vi "Swerve_Simple Config.vi"(11 "Module Azimuth Config Data":T7) -> (0 "PhoenixMotorControlDevRef Out":T2, 1 "PhoenixMotorControlDevRef Out":T2, 2 "CTRE_CANcoder_DeviceRef Out":T1, 3 "Motor Pos Out":T8)   [LabVIEW 2023, in "Thor-SwerveDrive_ACT.lvlib"]
uses:
  Thor-SwerveDrive_ACT.lvlib
  <vilib>/Rock Robotics/WPI/ThirdParty/Phoenix-LabVIEW/CANCoder/Set/CTRE_Phoenix_CANcoder_SetPositionToAbsolute.vi
  Shared Code/TypeDefs/ENUM_Motor Index.ctl
  Shared Code/TypeDefs/Cluster_Module Specific Config Data.ctl
  <vilib>/Rock Robotics/SystemInterfaces/DIO/FPGA_DIOPWMChannel.ctl
  <vilib>/Rock Robotics/WPI/PWM/WPI_PWMDeadband.ctl
  <vilib>/Rock Robotics/WPI/MotorControl/WPI_MotorControlType.ctl
  <vilib>/Rock Robotics/SystemInterfaces/DIO/FPGA_DIOChannel.ctl
  <vilib>/Rock Robotics/WPI/MotorControl/WPI_MotorControlDeviceRef.ctl
  <vilib>/Rock Robotics/WPI/ThirdParty/Phoenix-LabVIEW/CANCoder/Controls/CTRE_Phoenix_CANcoder_DeviceRef.ctl
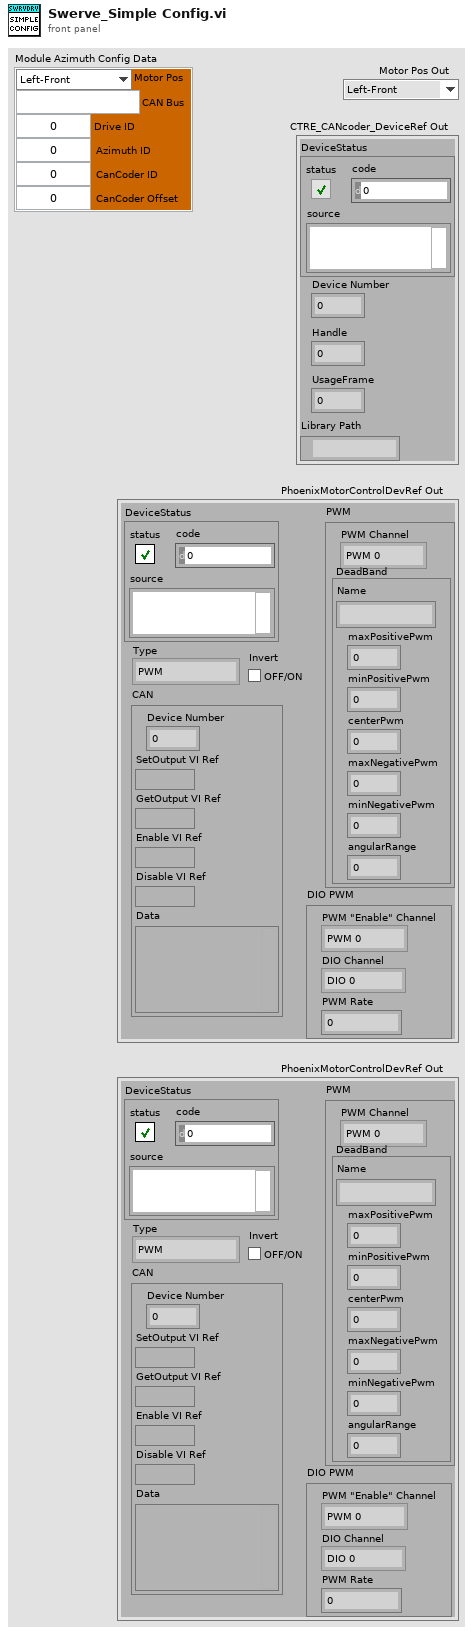
[diagram p1: front panel]
types:
  T1 = typedef "CTRE_Phoenix_CANcoder_DeviceRef.ctl" = cluster{"DeviceStatus":errorcluster, "Device Number":u8, "Handle":u64, "UsageFrame":u32, "Library Path":path}
  T2 = typedef "WPI_MotorControlDeviceRef.ctl" = cluster{"DeviceStatus":errorcluster, "Type":T3, "PWM":cluster{"PWM Channel":T4, "DeadBand":T5}, "CAN":cluster{"Device Number":u8, "SetOutput VI Ref":variant, "GetOutput VI Ref":variant, "Enable VI Ref":variant, "Disable VI Ref":variant, "Data":variant}, "Invert":bool, "DIO PWM":cluster{"PWM \"Enable\" Channel":T4, "DIOChannel":T6, "PWM Rate":dbl}}
  T3 = typedef "WPI_MotorControlType.ctl" = enum16{"PWM", "CAN", "DIO PWM"}
  T4 = typedef "FPGA_DIOPWMChannel.ctl" = enum8{"PWM 0", "PWM 1", "PWM 2", "PWM 3", "PWM 4", "PWM 5", "PWM 6", "PWM 7", "PWM 8", "PWM 9", "PWM MXP 0", "PWM MXP 1", "PWM MXP 2", "PWM MXP 3", "PWM MXP 4", "PWM MXP 5", "PWM MXP 6", "PWM MXP 7", "PWM MXP 8", "PWM MXP 9", "Invalid"}
  T5 = typedef "WPI_PWMDeadband.ctl" = cluster{"Name":string, "maxPositivePwm":i32, "minPositivePwm":i32, "centerPwm":i32, "maxNegativePwm":i32, "minNegativePwm":i32, "angularRange":u16}
  T6 = typedef "FPGA_DIOChannel.ctl" = enum8{"DIO 0", "DIO 1", "DIO 2", "DIO 3", "DIO 4", "DIO 5", "DIO 6", "DIO 7", "DIO 8", "DIO 9", "DIO MXP 0", "DIO MXP 1", "DIO MXP 2", "DIO MXP 3", "DIO MXP 4", "DIO MXP 5", "DIO MXP 6", "DIO MXP 7", "DIO MXP 8", "DIO MXP 9", "DIO MXP 10", "DIO MXP 11", "DIO MXP 12", "DIO MXP 13", "DIO MXP 14", "DIO MXP 15", "SPI Port CS1", "SPI Port CS2", "SPI Port CS3", "SPI Port MISO", "SPI Port MOSI", "Invalid"}
  T7 = typedef "Cluster_Module Specific Config Data.ctl" = cluster{"Motor Pos":T8, "CAN Bus":string, "Drive ID":u8, "Azimuth ID":u8, "CanCoder ID":u8, "CanCoder Offset":dbl}
  T8 = typedef "ENUM_Motor Index.ctl" = enum16{"Left-Front", "Right-Front", "Left-Back", "Right-Back"}
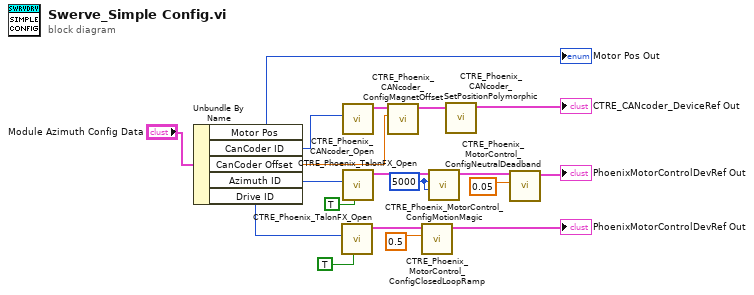
[diagram p0: block diagram]
diagram:
  w8 = 5000 ("Cruise Velocity")
  n1 = Unbundle By Name("Module Azimuth Config Data") -> ("Motor Pos"=→"Motor Pos Out":T8, "CanCoder ID"=w16:u8, "CanCoder Offset"=w1:dbl, "Azimuth ID"=w17:u8, "Drive ID"=w18:u8)
  n2 = call <vilib>:"CTRE_Phoenix_TalonFX_Open.vi"("Invert"=TRUE, "Device Number"=w18) -> ("PhoenixMotorControlDevRef"=w12:T2)  [unwired: 8 in, 1 out]
  n3 = call <vilib>:"CTRE_Phoenix_CANcoder_Open.vi"("Device Number"=w16) -> ("CTRE_CANcoder_DeviceRef"=w3:T1)  [unwired: 9 in, 1 out]
  n4 = call <vilib>:"CTRE_Phoenix_TalonFX_Open.vi"("Invert"=TRUE, "Device Number"=w17) -> ("PhoenixMotorControlDevRef"=w7:T2)  [unwired: 8 in, 1 out]
  n5 = call <vilib>:"CTRE_Phoenix_CANcoder_ConfigMagnetOffset.vi"("Magnet Offset (Degrees)"=w1, "CTRE_CANcoder_DeviceRef"=w3) -> ("CTRE_CANcoder_DeviceRef"=w4:T1)  [unwired: 8 in, 1 out]
  n6 = call <vilib>:"CTRE_Phoenix_MotorControl_ConfigClosedLoopRamp.vi"("secondsFromNeutralToFull"=0.5, "PhoenixMotorControlDevRef"=w12) -> ("PhoenixMotorControlDevRef"=→"PhoenixMotorControlDevRef Out":T2)  [unwired: 8 in, 1 out]
  n7 = call <vilib>:"CTRE_Phoenix_MotorControl_ConfigMotionMagic.vi"("Acceleration"=w8, "Cruise Velocity"=w8, "PhoenixMotorControlDevRef"=w7) -> ("PhoenixMotorControlDevRef"=w9:T2)  [unwired: 7 in, 1 out]
  n8 = call-poly <vilib>:"CTRE_Phoenix_CANcoder_SetPositionPolymorphic.vi"("CTRE_CANcoder_DeviceRef"=w4) -> ("CTRE_CANcoder_DeviceRef"=→"CTRE_CANcoder_DeviceRef Out":T1)  [unwired: 9 in, 1 out]
  n9 = call <vilib>:"CTRE_Phoenix_MotorControl_ConfigNeutralDeadband.vi"("Percent Deadband"=0.05, "PhoenixMotorControlDevRef"=w9) -> ("PhoenixMotorControlDevRef"=→"PhoenixMotorControlDevRef Out":T2)  [unwired: 8 in, 1 out]
